vi "Add To Project.vi"(8 "error in (no error)":errorcluster, 10 "References":T1) -> (0 "error out":errorcluster, 2 "Out":T1)   [LabVIEW 2023, in "Message Maker.lvclass"]
doc: "Adds the new message to the project\n\nAuthor: Derek Trepanier\nCopyright: MGI 2015"
uses:
  Message Maker.lvclass
  Message Maker.lvclass/Message Maker.ctl
  Scripting Refs.ctl
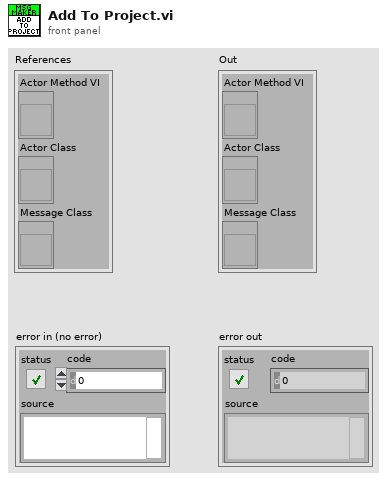
[diagram p1: front panel]
types:
  T1 = typedef "Message Maker.lvclass/Scripting Refs.ctl" = cluster{"Actor Method VI":refnum<vi>, "Actor Class":refnum<vi>, "Message Class":refnum<vi>}
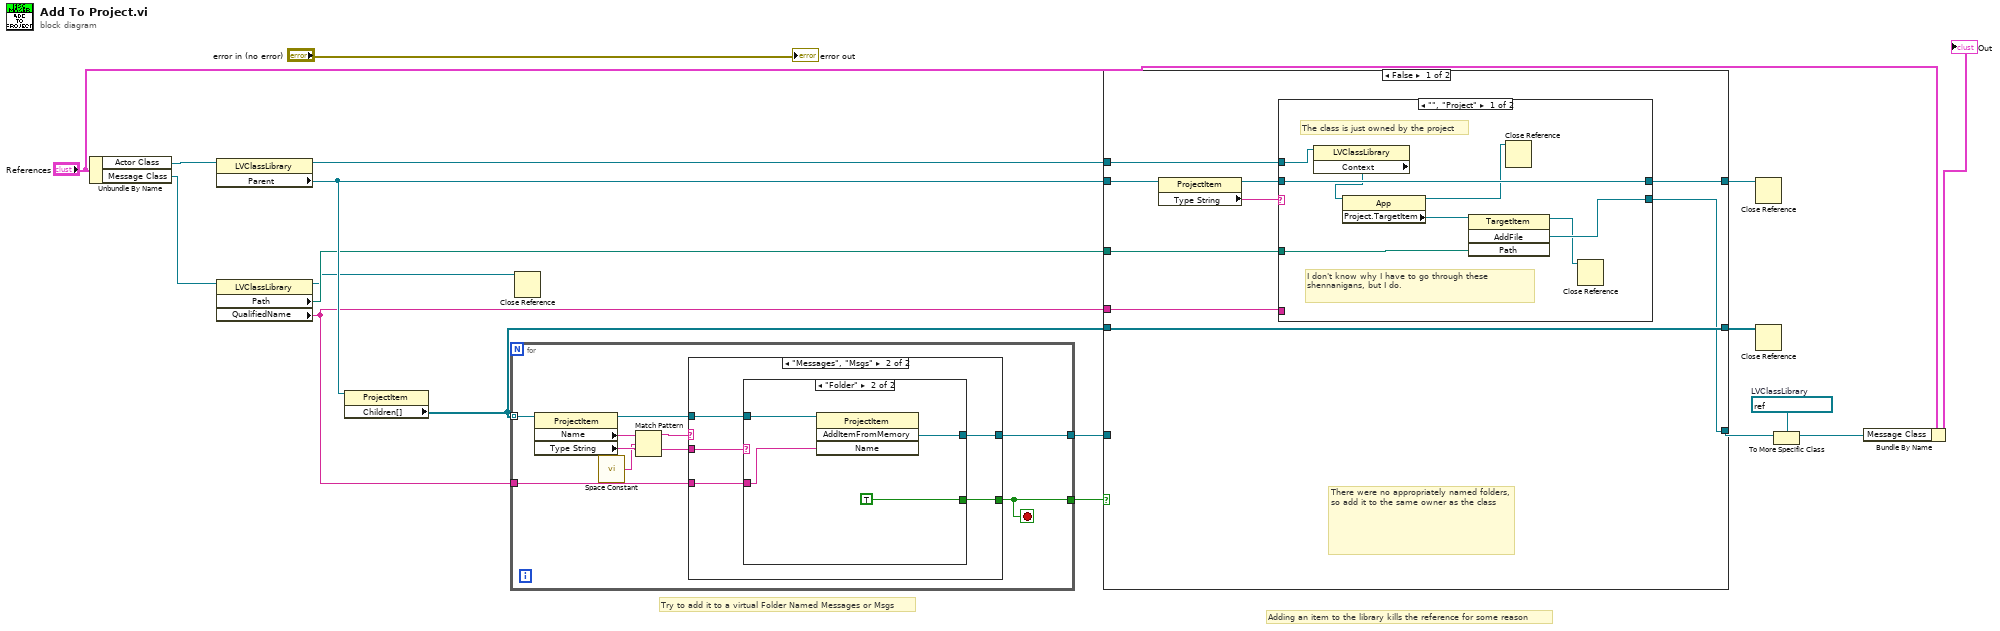
[diagram p0: block diagram]
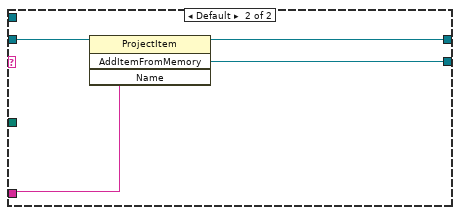
[diagram p2: hidden frame]
diagram:
  w6 = refnum<vi> refnum  # LVClassLibrary
  # "Adding an item to the library kills the reference for some reason"
  # "Try to add it to a virtual Folder Named Messages or Msgs"
  n1 = Unbundle By Name("References") -> ("Actor Class"=w18:refnum<vi>, "Message Class"=w17:refnum<vi>)
  n2 = property class="LVClassLibrary"(reference=w18) -> (reference out=w1:refnum<vi>, "Parent"=w14:refnum<vi>)  [unwired: 1 in, 1 out]
  n3 = property class="LVClassLibrary"(reference=w17) -> (reference out=w2:refnum<vi>, "Path"=w3:path, "QualifiedName"=w13:string)  [unwired: 1 in, 1 out]
  n4 = property class="ProjectItem"(reference=w14) -> ("Children[]"=w11:refnum<vi>[])  [unwired: 1 in, 2 out]
  n5 = for {
    tunnel: w11 -> [w25] mode=indexing
    tunnel: w13 -> [w26]
    tunnel: [w22] -> w15
    tunnel: [w23] -> w8
    stop <- w22 stop-if-true
    n6 = property class="ProjectItem"(reference=w25) -> (reference out=w27:refnum<vi>, "Name"=w21:string, "Type String"=w24:string)  [unwired: 1 in, 1 out]
    n7 = call <vilib>:"Space Constant.vi"() -> ("String"=w19:string)
    n8 = Match Pattern(string=w21, regular expression=w19) -> (before substring=w20:string)  [unwired: 1 in, 3 out]
    n9 = case shown="\"Messages\", \"Msgs\"" w20 {
      tunnel: w27 -> [_ w32]
      tunnel: w26 -> [_ w31]
      tunnel: [_ w30] -> w22
      tunnel: w24 -> [_ w29]
      tunnel: [_ w28] -> w23
      frame Default {
      }
      frame "Messages", "Msgs" {
        n10 = case shown="\"Folder\"" w29 {
          tunnel: w32 -> [_ w36]
          tunnel: w31 -> [_ w34]
          tunnel: [_ TRUE] -> w30
          tunnel: [_ w33] -> w28
          frame Default {
          }
          frame "Folder" {
            n11 = invoke class="ProjectItem" method="AddItemFromMemory"(reference=w36, "Name"=w34) -> ("AddItemFromMemory"=w33:refnum<vi>)  [unwired: 2 in, 3 out]
          }
        }
      }
    }
  }
  n12 = Close Reference(reference=w2) -> ()  [unwired: 1 in, 1 out]
  n13 = case shown="False" w15 {
    tunnel: w14 -> [w41 w60]
    tunnel: w13 -> [w45 _]
    tunnel: [w44 w60] -> w12
    tunnel: w11 -> [w43 w59]
    tunnel: [w43 w59] -> w10
    tunnel: w8 -> [_ w58]
    tunnel: [w42 w58] -> w7
    tunnel: w3 -> [w38 _]
    tunnel: w1 -> [w37 _]
    frame False {
      # "There were no appropriately named folders, so add it to the same owner as the class"
      n14 = property class="ProjectItem"(reference=w41) -> (reference out=w40:refnum<vi>, "Type String"=w39:string)  [unwired: 1 in, 1 out]
      n15 = case shown="\"\", \"Project\"" w39 {
        tunnel: w45 -> [_ w57]
        tunnel: [w53 w56] -> w44
        tunnel: [w51 w55] -> w42
        tunnel: w40 -> [w53 w54]
        tunnel: w38 -> [w52 _]
        tunnel: w37 -> [w50 _]
        frame "", "Project" {
          # "I don't know why I have to go through these shennanigans, but I do."
          # "The class is just owned by the project"
          n16 = property class="LVClassLibrary"(reference=w50) -> ("Context"=w49:refnum<vi>)  [unwired: 1 in, 2 out]
          n17 = property class="App"(reference=w49) -> (reference out=w46:refnum<vi>, "Project.TargetItem"=w48:refnum<vi>)  [unwired: 1 in, 1 out]
          n18 = invoke class="TargetItem" method="AddFile"(reference=w48, "Path"=w52) -> (reference out=w47:refnum<vi>, "AddFile"=w51:refnum<vi>)  [unwired: 2 in, 2 out]
          n19 = Close Reference(reference=w46) -> ()  [unwired: 1 in, 1 out]
          n20 = Close Reference(reference=w47) -> ()  [unwired: 1 in, 1 out]
        }
        frame Default {
          n21 = invoke class="ProjectItem" method="AddItemFromMemory"(reference=w54, "Name"=w57) -> (reference out=w56:refnum<vi>, "AddItemFromMemory"=w55:refnum<vi>)  [unwired: 2 in, 2 out]
        }
      }
    }
    frame True {
    }
  }
  n22 = Close Reference(reference=w12) -> ()  [unwired: 1 in, 1 out]
  n23 = Close Reference(reference=w10) -> ()  [unwired: 1 in, 1 out]
  n24 = To More Specific Class(target class=w6, reference=w7) -> (specific class reference=w4:refnum<vi>)  [unwired: 1 in, 1 out]
  n25 = Bundle By Name(cluster="References", "Message Class"=w4) -> (→"Out":T1)
  "error out" <- "error in (no error)"
